vi "Module Set Instance.vi"(8 "error in (no error)":errorcluster, 10 "Instance":T1, 11 "Self in":variant) -> (0 "error out":errorcluster, 3 "Self out":variant)   [LabVIEW 2018, in "Core.lvlib"]
uses:
  Core.lvlib
  Controls/Module Instance.ctl
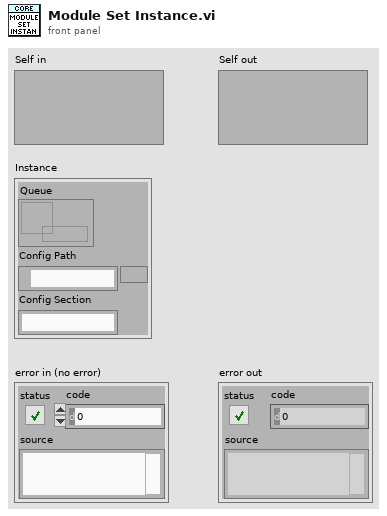
[diagram p1: front panel]
types:
  T1 = typedef "Core.lvlib/Module Instance.ctl" = cluster{"Queue":refnum<queue>, "Config Path":path, "Config Section":string}
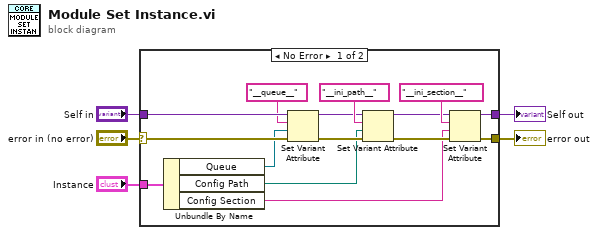
[diagram p0: block diagram]
diagram:
  n1 = case shown="No Error" "error in (no error)" {
    selector: "error in (no error)" -> [w20 w22]
    tunnel: "Self in" -> [w19 w21]
    tunnel: "Instance" -> [w18 _]
    tunnel: [w7 w22] -> w2
    tunnel: [w6 w21] -> w1
    frame No Error {
      n2 = Unbundle By Name(w18) -> ("Queue"=w16:refnum<queue>, "Config Path"=w12:path, "Config Section"=w8:string)
      n3 = Set Variant Attribute(Variant=w19, name="__queue__", value=w16, error in=w20) -> (Variant out=w14:variant, error out=w13:errorcluster)  [unwired: 1 out]
      n4 = Set Variant Attribute(Variant=w14, name="__ini_path__", value=w12, error in=w13) -> (Variant out=w10:variant, error out=w9:errorcluster)  [unwired: 1 out]
      n5 = Set Variant Attribute(Variant=w10, name="__ini_section__", value=w8, error in=w9) -> (Variant out=w6:variant, error out=w7:errorcluster)  [unwired: 1 out]
    }
    frame Error {
    }
  }
  "Self out" <- w1
  "error out" <- w2
